vi "Peek Stream.vi"(8 "error in (no error)":errorcluster, 10 "timeout in ms (-1)":i32, 11 "stream in":refnum<queue>) -> (0 "error out":errorcluster, 2 "element":T1, 3 "queue out":refnum<queue>)   [LabVIEW 2014, in "Sprocket.lvlib"]
uses:
  lib/Sprocket.lvlib
  Action/Action.ctl
  Action/Action Name.ctl
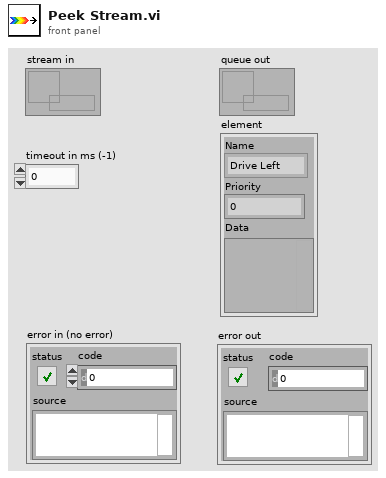
[diagram p1: front panel]
types:
  T1 = typedef "Sprocket.lvlib/Action.ctl" = cluster{"Name":T2, "Priority":i32, "Data":variant}
  T2 = typedef "Sprocket.lvlib/Action Name.ctl" = enum16{"Drive Left", "Drive Right"}
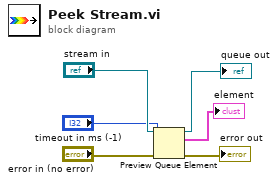
[diagram p0: block diagram]
diagram:
  n1 = Preview Queue Element(queue="stream in", timeout in ms (-1)="timeout in ms (-1)", error in (no error)="error in (no error)") -> (queue out=→"queue out":refnum<queue>, element=→"element":T1, error out=→"error out":errorcluster)  [unwired: 1 out]
